vi "Get All Values.vi"(8 "error in (no error)":errorcluster, 11 "Keyed Value Tree in":refnum<class "Keyed Value Tree.lvclass">) -> (0 "error out":errorcluster, 2 "Keyed Value Pairs":T1[](array[typedef]), 3 "Keyed Value Tree out":refnum<class "Keyed Value Tree.lvclass">)   [LabVIEW 2027, in "Keyed Value Tree.lvclass"]
uses:
  Keyed Value Tree.lvclass
  Keyed Value Pair.ctl
  Keyed Value Tree.lvclass/Keyed Value Tree.ctl
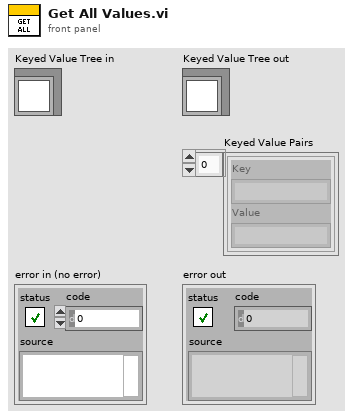
[diagram p1: front panel]
types:
  T1 = typedef "Keyed Value Tree.lvclass/Keyed Value Pair.ctl" = cluster{"Key":string, "Value":string}
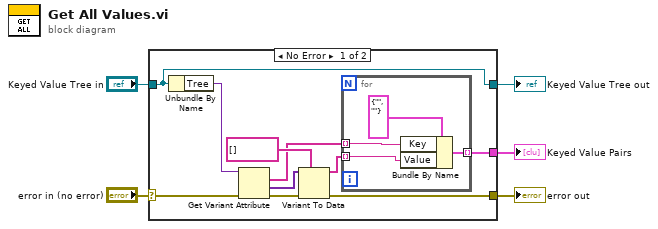
[diagram p0: block diagram]
diagram:
  n1 = case shown="No Error" "error in (no error)" {
    selector: "error in (no error)" -> [w8 w21]
    tunnel: [w6 w21] -> w4
    tunnel: [w15 w20] -> w2
    tunnel: "Keyed Value Tree in" -> [w15 w20]
    tunnel: [w9 _] -> w1
    frame No Error {
      n2 = Unbundle By Name(w15) -> ("Tree"=w14:variant)
      n3 = Get Variant Attribute(Variant=w14, error in=w8) -> (names=w11:string[], values=w13:variant[], error out=w7:errorcluster)  [unwired: 2 in, 1 out]
      n4 = Variant To Data(error in=w7, type=string[] [], Variant=w13) -> (data=w10:string[], error out=w6:errorcluster)
      n5 = for {
        tunnel: w11 -> [w18] mode=indexing
        tunnel: w10 -> [w17] mode=indexing
        tunnel: [w16] -> w9 mode=indexing
        n6 = Bundle By Name(cluster=T1 {"Key"="", "Value"=""} ("KVP"), "Key"=w18, "Value"=w17) -> (w16:T1)
      }
    }
    frame Error {
    }
  }
  "error out" <- w4
  "Keyed Value Tree out" <- w2
  "Keyed Value Pairs" <- w1
